vi "sendCommandL1Test.vi"() -> ()   [LabVIEW 2009]
uses:
  <vilib>/Utility/NIReport.llb/NI_report.lvclass
  <vilib>/Utility/NIReport.llb/HTML/NI_HTML.lvclass
panel:
  out "bytes written":i32
  in  "Address":i32
  in  "Data":i32
  out "Data out":string
  out "Instrument VISA out":T1={"AWG VISA"="generadorpulsos", "Oscilloscope  VISA "="Oscilloscope", "Integration Board IP"="172.16.7.43", "connection ID"=refnum, "report out"=refnum, "report file path"=path "C:/Documents and Settings/CTA_LAB01/Desktop/L0_Asic/L0 Asic Test Data"}
  out "error out":errorcluster
  in  "Instrument VISA in":T1={"AWG VISA"="generadorpulsos", "Oscilloscope  VISA "="Oscilloscope", "Integration Board IP"="172.16.7.43", "connection ID"=refnum, "report out"=refnum, "report file path"=path "C:/Documents and Settings/CTA_LAB01/Desktop/L0_Asic/L0 Asic Test Data"}
  in  "error in (no error)":errorcluster
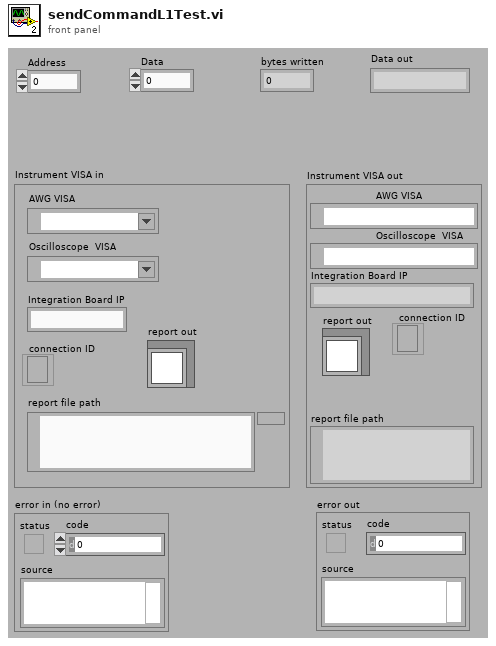
[diagram p1: front panel]
types:
  T1 = cluster{"AWG VISA":refnum<visa-resource-name>, "Oscilloscope  VISA ":refnum<visa-resource-name>, "Integration Board IP":string, "connection ID":refnum<k5>, "report out":refnum<class "NI_report.lvclass">, "report file path":path}
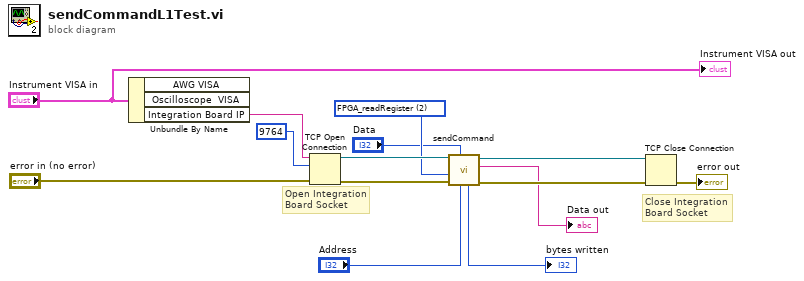
[diagram p0: block diagram]
diagram:
  w5 = u16 2 items=["sendCommand"=9, "FPGA_writeRegister"=3, "FPGA_readRegister"=2, "uC_writeRegister"=1, "uC_readRegister"=0] ("Action")
  # "Close Integration \nBoard Socket"
  # "Open Integration\nBoard Socket"
  n1 = Unbundle By Name("Instrument VISA in") -> ("Integration Board IP"=w13:string)  [unwired: 2 out]
  n2 = TCP Open Connection(address=w13, remote port or service name=9764, error in (no error)="error in (no error)") -> (connection ID=w11:refnum<k5>, error out=w10:errorcluster)  [unwired: 2 in]
  n3 = call "sendCommand.vi"("Address"="Address", "Data"="Data", "error in"=w10, "Action"=w5, "connection ID"=w11) -> ("error out"=w8:errorcluster, "Data out"=→"Data out":string, "connection ID out"=w7:refnum<k5>, "bytes written"=→"bytes written":i32)  [unwired: 2 in, 1 out]
  n4 = TCP Close Connection(connection ID=w7, error in (no error)=w8) -> (error out=→"error out":errorcluster)  [unwired: 1 in, 1 out]
  "Instrument VISA out" <- "Instrument VISA in"
